vi "Replace BD Constant.vi"(8 "error in (no error)":errorcluster, 11 "Setter Generator In":refnum<class "Setter Generator.lvclass">) -> (0 "error out":errorcluster, 3 "Setter Generator Out":refnum<class "Setter Generator.lvclass">)   [LabVIEW 2020, in "Method Generation.lvlib" / "Setter Generator.lvclass"]
uses:
  Setter Generator.lvclass
  <vilib>/Utility/traverseref.llb/TRef TravTarget.ctl
  Setter Generator.lvclass/Setter Generator.ctl
  <vilib>/Utility/traverseref.llb/VI Scripting - Traverse.lvlib
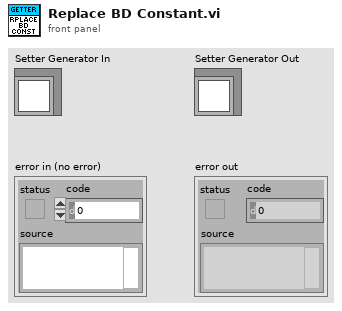
[diagram p1: front panel]
types:
  T1 = typedef "TRef TravTarget.ctl" = enum16{"FP", "BD", "Other"}
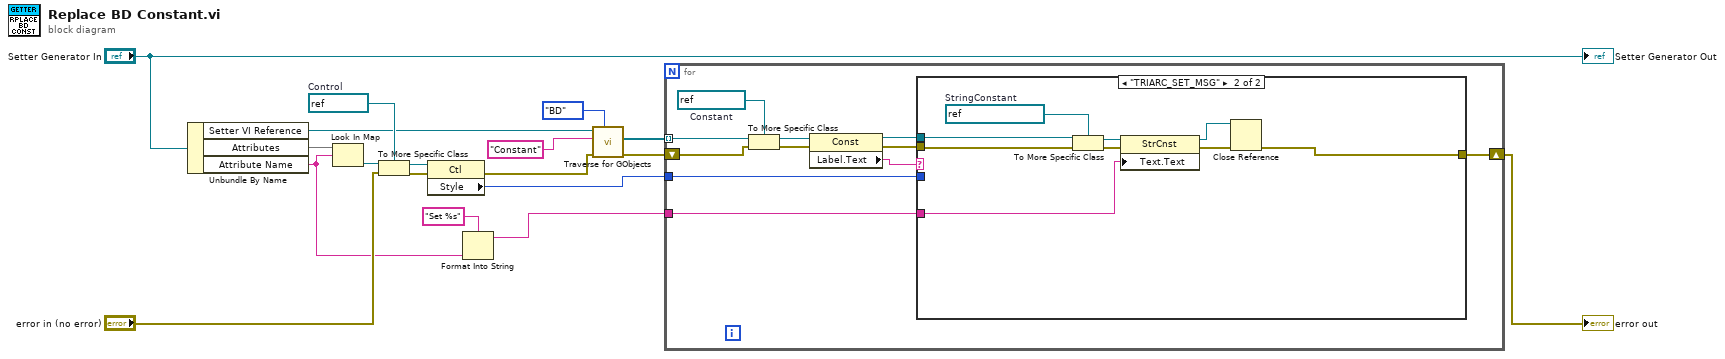
[diagram p0: block diagram]
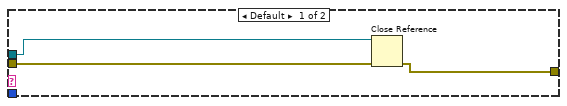
[diagram p2: hidden frame]
diagram:
  w13 = refnum<vi> refnum  # Control
  n1 = Unbundle By Name("Setter Generator In") -> ("Setter VI Reference"=w4:refnum<vi>, "Attributes"=w16:map{string, refnum<vi>}, "Attribute Name"=w6:string)
  n2 = Look In Map(map=w16, key=w6) -> (value=w15:refnum<vi>)  [unwired: 1 in, 1 out]
  n3 = To More Specific Class(target class=w13, reference=w15, error in="error in (no error)") -> (specific class reference=w14:refnum<vi>, error out=w11:errorcluster)
  n4 = property class="Ctl"(reference=w14, error in=w11) -> (error out=w9:errorcluster, "Style"=w12:u32)  [unwired: 1 out]
  n5 = Format Into String(format string="Set %s", w6) -> (resulting string=w5:string)  [unwired: 2 in, 1 out]
  n6 = call <vilib>:"Traverse for GObjects.vi"("Traverse Target"=TRef_TravTarget."BD", "error in (no error)"=w9, "Class Name"="Constant", "VI Refnum"=w4) -> ("error out"=w2:errorcluster, "References"=w3:refnum<vi>[])  [unwired: 4 in, 2 out]
  n7 = for {
    tunnel: w3 -> [w29] mode=indexing
    tunnel: w12 -> [w27]
    shift-right: [w26] -> w1
    shift-left: w2 -> [w28]
    tunnel: w5 -> [w19]
    w25 = refnum<vi> refnum  # Constant
    n8 = To More Specific Class(target class=w25, reference=w29, error in=w28) -> (specific class reference=w22:refnum<vi>, error out=w24:errorcluster)
    n9 = property class="Const"(reference=w22, error in=w24) -> (reference out=w21:refnum<vi>, error out=w23:errorcluster, "Label.Text"=w20:string)
    n10 = case shown="\"TRIARC_SET_MSG\"" w20 {
      tunnel: w27 -> [_ _]
      tunnel: [w31 w34] -> w26
      tunnel: w23 -> [w32 w40]
      tunnel: w21 -> [w30 w41]
      tunnel: w19 -> [_ w36]
      frame Default {
        n11 = Close Reference(reference=w30, error in (no error)=w32) -> (error out=w31:errorcluster)
      }
      frame "TRIARC_SET_MSG" {
        w39 = refnum<vi> refnum  # StringConstant
        n12 = To More Specific Class(target class=w39, reference=w41, error in=w40) -> (specific class reference=w38:refnum<vi>, error out=w37:errorcluster)
        n13 = property class="StrCnst"(reference=w38, error in=w37, "Text.Text"=w36) -> (reference out=w33:refnum<vi>, error out=w35:errorcluster)
        n14 = Close Reference(reference=w33, error in (no error)=w35) -> (error out=w34:errorcluster)
      }
    }
  }
  "error out" <- w1
  "Setter Generator Out" <- "Setter Generator In"
